vi "Initialize.vi"(8 "error in (no error)":errorcluster, 11 "IMAQ Camera in":refnum<class "IMAQ Camera.lvclass">) -> (0 "error out":errorcluster, 3 "IMAQ Camera out":refnum<class "IMAQ Camera.lvclass">)   [LabVIEW 2011, in "IMAQ Camera.lvclass"]
uses:
  IMAQ Camera.lvclass
  Camera Class/Camera.lvclass
  IMAQ Camera.lvclass/IMAQ Camera.ctl
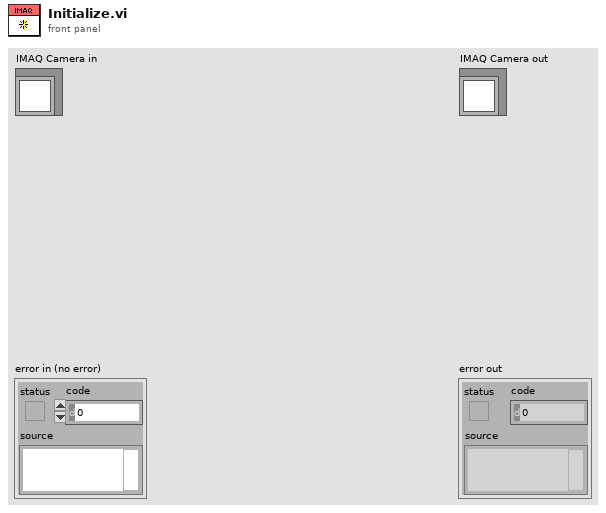
[diagram p1: front panel]
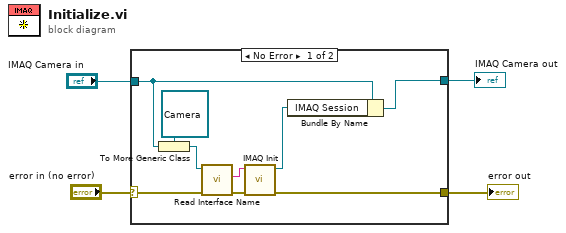
[diagram p0: block diagram]
diagram:
  n1 = case shown="No Error" "error in (no error)" {
    selector: "error in (no error)" -> [w5 w14]
    tunnel: "IMAQ Camera in" -> [w9 w15]
    tunnel: [w7 w15] -> w3
    tunnel: [w6 w14] -> w2
    frame No Error {
      n2 = To More Generic Class(target class=refnum<class "Camera.lvclass"> refnum ("Image UDP Broadcast Custom Device.lvlib:Camera.lvclass"), reference=w9) -> (generic class reference=w12:refnum<class "Camera.lvclass">)
      n3 = call-dynamic "Read Interface Name.vi"("error in (no error)"=w5, "Camera in"=w12) -> ("error out"=w10:errorcluster, "Interface Name"=w11:string)  [unwired: 7 in, 1 out]
      n4 = call <vilib>:"IMAQ Init.vi"("error in (no error)"=w10, "Interface Name"=w11) -> ("error out"=w6:errorcluster, "IMAQ Session Out"=w8:refnum<k11>)  [unwired: 8 in]
      n5 = Bundle By Name(cluster=w9, "IMAQ Session"=w8) -> (w7:refnum<class "IMAQ Camera.lvclass">)
    }
    frame Error {
    }
  }
  "error out" <- w2
  "IMAQ Camera out" <- w3
